vi "Initialize Entry.vi"(6 "chip select (1st chip)":enum16{"1st chip", "2nd chip"}(ring), 8 "error in (no error)":errorcluster, 11 "HD44780 in":refnum<class "HD44780.lvclass">) -> (0 "error out":errorcluster, 3 "HD44780 out":refnum<class "HD44780.lvclass">)   [LabVIEW 2017, in "HD44780.lvclass"]
uses:
  HD44780.lvclass
  HD44780.lvclass/HD44780.ctl
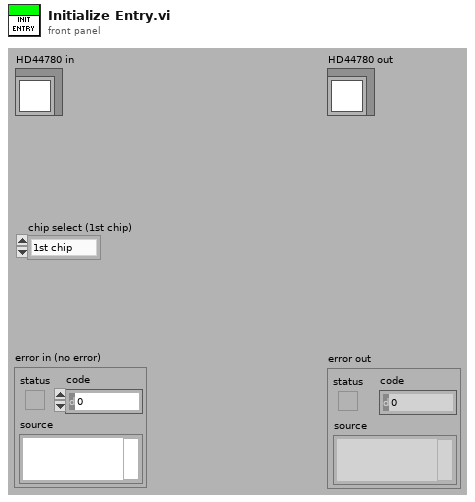
[diagram p1: front panel]
types:
  T1 = typedef "HD44780 Common.lvlib/cluster of class private data.ctl" = cluster{"FPGA VI Reference":refnum<k20>, "device index":i8, "screen size":T2, "font size":T3, "auto wrap":bool, "alignment":T4, "number of line":T5, "shift 0":i8, "entry mode 0":T6, "shift 1":i8, "entry mode 1":T6}
  T2 = typedef "HD44780 Common.lvlib/screen size.ctl" = enum8{"8x1", "8x2", "12x4", "16x1", "16x2", "16x4", "20x1", "20x2", "20x4", "24x1", "24x2", "40x2", "40x4"}
  T3 = typedef "HD44780 Common.lvlib/font size.ctl" = enum8{"5x8", "5x10"}
  T4 = typedef "HD44780 Common.lvlib/alignment.ctl" = enum16{"None", "Left", "Center", "Right"}
  T5 = typedef "HD44780 Common.lvlib/line number.ctl" = enum8{"1 line", "2 lines"}
  T6 = typedef "HD44780 Common.lvlib/entry mode.ctl" = enum8{"increment & no shift", "increment & shift", "decrement & no shift", "decrement & shift"}
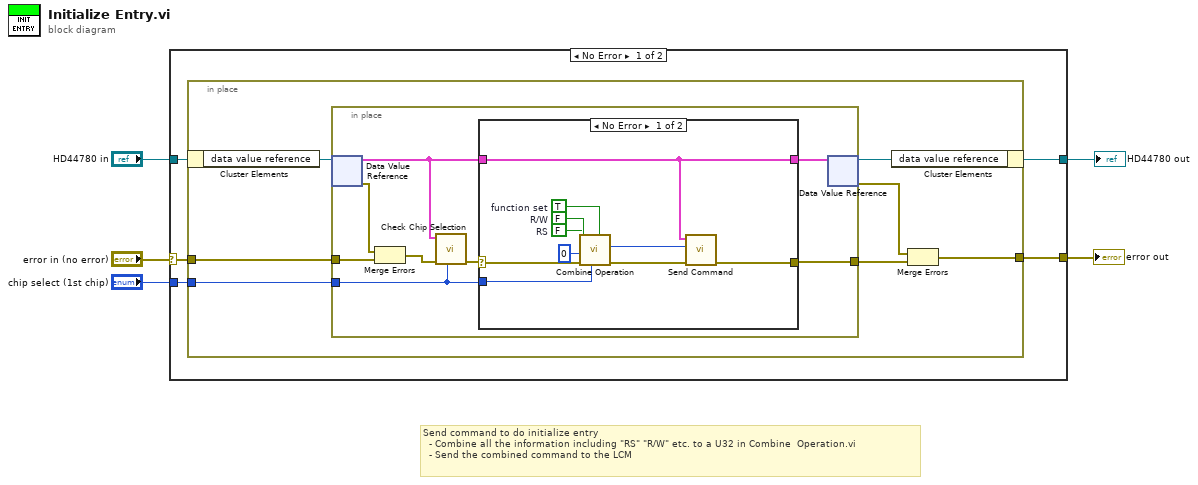
[diagram p0: block diagram]
diagram:
  # "Send command to do initialize entry\n  - Combine all the information including \"RS\" \"R/W\" etc. to a U32 in Combine  Operation.vi \n  - Send the combined command to the LCM"
  n1 = case shown="No Error" "error in (no error)" {
    selector: "error in (no error)" -> [w6 w38]
    tunnel: [w10 w38] -> w5
    tunnel: "chip select (1st chip)" -> [w9 _]
    tunnel: "HD44780 in" -> [w8 w39]
    tunnel: [w7 w39] -> w2
    frame No Error {
      n2 = in-place {
        in-place-border: [w12] -> w10
        in-place-border: w9 -> [w17]
        in-place-border: w6 -> [w11]
        n3 = in-place-cluster #1(w8) -> ("data value reference"=w16:refnum<data-value>)
        n4 = in-place {
          in-place-border: [w25] -> w13
          in-place-border: w17 -> [w18]
          in-place-border: w11 -> [w19]
          n5 = in-place-dvr #2(w16) -> (w23:T1, w20:errorcluster)
          n6 = Merge Errors(w20, w19) -> (w21:errorcluster)
          n7 = call "Check Chip Selection.vi"("chip select"=w18, "error in (no error)"=w21, "cluster of private data in"=w23) -> ("error out"=w24:errorcluster)  [unwired: 7 in, 1 out]
          n8 = case shown="No Error" w24 {
            selector: w24 -> [w30 w37]
            tunnel: [w33 w37] -> w25
            tunnel: w18 -> [w29 _]
            tunnel: w23 -> [w27 w36]
            tunnel: [w27 w36] -> w22
            frame No Error {
              w26 = FALSE  # RS
              w31 = TRUE  # function set
              w35 = FALSE  # R/W
              n9 = call "Combine Operation.vi"("initialize entry (F)"=w31, "chip select  (1st chip)"=w29, "error in (no error)"=w30, "cmd/data"=u8 0, "RS"=w26, "R/W"=w35) -> ("error out"=w34:errorcluster, "output"=w28:u32)  [unwired: 4 in]
              n10 = call "Send Command.vi"("error in (no error)"=w34, "operation"=w28, "cluster of private data in"=w27) -> ("error out"=w33:errorcluster)  [unwired: 6 in, 2 out]
            }
            frame Error {
            }
          }
          n11 = in-place-dvr #2(w22) -> (w15:refnum<data-value>, w14:errorcluster)
        }
        n12 = in-place-cluster #1("data value reference"=w15) -> (w7:refnum<class "HD44780.lvclass">)
        n13 = Merge Errors(w14, w13) -> (w12:errorcluster)
      }
    }
    frame Error {
    }
  }
  "HD44780 out" <- w2
  "error out" <- w5
